vi "rsidr_core_global.vi"() -> ()   [LabVIEW 2020, in "Rohde&Schwarz CMWXP NR FR1 Measurement.lvlib"] (continued)
emission measurements exceeding the specified spectrum emission mask limits.\nDefault unit:  % \n\n<MarginX>\n float\nX-position of the margin of an area\nDefault unit:  Hz \n\n<MarginY>\n float\nY-value of the margin of an area\nDefault unit:  dB\n\nAvailable Repeated Capabilities:\ninstance: i0, i1, i2, i3, i4, i5, i6, i7, i8, i9, i10, i11, i12, i13, i14, i15, i16, i17, i18, i19, i20, i21, i22, i23, i24, i25, i26, i27, i28, i29, i30, i31, i32\r\n\nRemote-control command(s):\nFETCh:NRSub:MEAS<i>:MEValuation:SEMask:MARGin:MINimum:NEGativ?"}, {"Level"=4, "Class Only"=FALSE, "Identifier"="RSCMWXPNRFR1M_ATTR_FETCH_MULTI_EVAL_MEAS_SEM_MARGIN_ALL_RESULTS", "Descriptive Name"="Fetch Multi Eval Meas SEM Margin All Results", "Data Type"=enum."RawString", "Command"="FETC:NRS:MEAS{instance}:MEV:SEM:MARG:ALL?", "Access"=enum."Read Only", "Range Table"="", "Read Callback"="", "Write Callback"="", "Range Callback"="", "Check Callback"="", "Rngtable Callback"="", "Coerce Callback"="", "Supported Models"="", "Instrument Options"="", "Check Status Callback"="", "Flags"=0, "Help"="Returns spectrum emission mask margin results. A negative margin indicates that the trace is located above the limit line, i.e. the limit is exceeded. Results are provided for the current, average and maximum traces. For each trace, 24 values related to the negative (Neg) and positive (Pos) offset frequencies of emission mask areas 1 to 12 are provided. For inactive areas, NCAP is returned.\n\nReturn values:  \n<1_Reliability>\n decimal\n\n<2_OutOfTol>\n decimal\nOut of tolerance result, i.e. percentage of measurement intervals of the statistic count for spectrum emission measurements exceeding the specified spectrum emission mask limits.\nDefault unit:  % \n\n<3_CurrNeg1> ... <14_CurrNeg12>\n float\nMargin results for current trace, negative offsets\nDefault unit:  dB \n\n<15_CurrPos1> ... <26_CurrPos12>\n float\nMargin results for current trace, positive offsets\nDefault unit:  dB \n\n<27_AvgNeg1> ... <38_AvgNeg12>\n float\nMargin results for average trace, negative offsets\nDefault unit:  dB \n\n<39_AvgPos1> ... <50_AvgPos12>\n float\nMargin results for average trace, positive offsets\nDefault unit:  dB \n\n<51_MinNeg1> ... <62_MinNeg12>\n float\nMargin results for maximum trace (resulting in minimum margins), negative offsets\nDefault unit:  dB \n\n<63_MinPos1> ... <74_MinPos12>\n float\nMargin results for maximum trace (resulting in minimum margins), positive offsets\nDefault unit:  dB\n\nAvailable Repeated Capabilities:\ninstance: i0, i1, i2, i3, i4, i5, i6, i7, i8, i9, i10, i11, i12, i13, i14, i15, i16, i17, i18, i19, i20, i21, i22, i23, i24, i25, i26, i27, i28, i29, i30, i31, i32\r\n\nRemote-control command(s):\nFETCh:NRSub:MEAS<i>:MEValuation:SEMask:MARGin:ALL?"}, {"Level"=4, "Class Only"=TRUE, "Identifier"="", "Descriptive Name"="RBW Trace", "Data Type"=enum."ViInt32", "Command"="", "Access"=enum."Read Only", "Range Table"="", "Read Callback"="", "Write Callback"="", "Range Callback"="", "Check Callback"="", "Rngtable Callback"="", "Coerce Callback"="", "Supported Models"="", "Instrument Options"="", "Check Status Callback"="", "Flags"=0, "Help"="This class contains commands to fetch trace results for the individual resolution bandwidths."}, {"Level"=5, "Class Only"=FALSE, "Identifier"="RSCMWXPNRFR1M_ATTR_READ_MULTI_EVAL_MEAS_SEM_TRACE_RBW_CURRENT_RESULTS", "Descriptive Name"="Read Multi Eval Meas SEM Trace RBW Current Results", "Data Type"=enum."RawString", "Command"="READ:NRS:MEAS{instance}:MEV:TRAC:SEM:RBW{RBW}:CURR?", "Access"=enum."Read Only", "Range Table"="", "Read Callback"="", "Write Callback"="", "Range Callback"="", "Check Callback"="", "Rngtable Callback"="", "Coerce Callback"="", "Supported Models"="", "Instrument Options"="", "Check Status Callback"="", "Flags"=0, "Help"="Returns the values of the spectrum emission traces. Separate traces are available for the individual resolution bandwidths (<kHz>). The results of the current trace are returned.\n\nReturn values:\n<Reliability>\n decimal\n\n<Power>\n float\nComma-separated list of power results\nThe value in the middle of the result array corresponds to the center frequency. The test point separation between two results depends on the resolution bandwidth. If there is no result for a frequency because no limit is defined, INV is returned.\nDefault unit:  dBm\n\nAvailable Repeated Capabilities:\ninstance: i0, i1, i2, i3, i4, i5, i6, i7, i8, i9, i10, i11, i12, i13, i14, i15, i16, i17, i18, i19, i20, i21, i22, i23, i24, i25, i26, i27, i28, i29, i30, i31, i32\r\nRBW: kHz30, kHz100, MHz1, BW1Pc, BW2Pc\r\n\nRemote-control command(s):\nREAD:NRSub:MEAS<i>:MEValuation:TRACe:SEMask:RBW<kHz>:CURRent?"}, {"Level"=5, "Class Only"=FALSE, "Identifier"="RSCMWXPNRFR1M_ATTR_READ_MULTI_EVAL_MEAS_SEM_TRACE_RBW_AVERAGE_RESULTS", "Descriptive Name"="Read Multi Eval Meas SEM Trace RBW Average Results", "Data Type"=enum."RawString", "Command"="READ:NRS:MEAS{instance}:MEV:TRAC:SEM:RBW{RBW}:AVER?", "Access"=enum."Read Only", "Range Table"="", "Read Callback"="", "Write Callback"="", "Range Callback"="", "Check Callback"="", "Rngtable Callback"="", "Coerce Callback"="", "Supported Models"="", "Instrument Options"="", "Check Status Callback"="", "Flags"=0, "Help"="Returns the values of the spectrum emission traces. Separate traces are available for the individual resolution bandwidths (<kHz>). The results of the average trace are returned.\n\nReturn values:\n<Reliability>\n decimal\n\n<Power>\n float\nComma-separated list of power results\nThe value in the middle of the result array corresponds to the center frequency. The test point separation between two results depends on the resolution bandwidth. If there is no result for a frequency because no limit is defined, INV is returned.\nDefault unit:  dBm\n\nAvailable Repeated Capabilities:\ninstance: i0, i1, i2, i3, i4, i5, i6, i7, i8, i9, i10, i11, i12, i13, i14, i15, i16, i17, i18, i19, i20, i21, i22, i23, i24, i25, i26, i27, i28, i29, i30, i31, i32\r\nRBW: kHz30, kHz100, MHz1, BW1Pc, BW2Pc\r\n\nRemote-control command(s):\nREAD:NRSub:MEAS<i>:MEValuation:TRACe:SEMask:RBW<kHz>:AVERage?"}, {"Level"=5, "Class Only"=FALSE, "Identifier"="RSCMWXPNRFR1M_ATTR_READ_MULTI_EVAL_MEAS_SEM_TRACE_RBW_MAXIMUM_RESULTS", "Descriptive Name"="Read Multi Eval Meas SEM Trace RBW Maximum Results", "Data Type"=enum."RawString", "Command"="READ:NRS:MEAS{instance}:MEV:TRAC:SEM:RBW{RBW}:MAX?", "Access"=enum."Read Only", "Range Table"="", "Read Callback"="", "Write Callback"="", "Range Callback"="", "Check Callback"="", "Rngtable Callback"="", "Coerce Callback"="", "Supported Models"="", "Instrument Options"="", "Check Status Callback"="", "Flags"=0, "Help"="Returns the values of the spectrum emission traces. Separate traces are available for the individual resolution bandwidths (<kHz>). The results of the maximum trace are returned.\n\nReturn values:\n<Reliability>\n decimal\n\n<Power>\n float\nComma-separated list of power results\nThe value in the middle of the result array corresponds to the center frequency. The test point separation between two results depends on the resolution bandwidth. If there is no result for a frequency because no limit is defined, INV is returned.\nDefault unit:  dBm\n\nAvailable Repeated Capabilities:\ninstance: i0, i1, i2, i3, i4, i5, i6, i7, i8, i9, i10, i11, i12, i13, i14, i15, i16, i17, i18, i19, i20, i21, i22, i23, i24, i25, i26, i27, i28, i29, i30, i31, i32\r\nRBW: kHz30, kHz100, MHz1, BW1Pc, BW2Pc\r\n\nRemote-control command(s):\nREAD:NRSub:MEAS<i>:MEValuation:TRACe:SEMask:RBW<kHz>:MAXimum?"}, {"Level"=5, "Class Only"=FALSE, "Identifier"="RSCMWXPNRFR1M_ATTR_FETCH_MULTI_EVAL_MEAS_SEM_TRACE_RBW_CURRENT_RESULTS", "Descriptive Name"="Fetch Multi Eval Meas SEM Trace RBW Current Results", "Data Type"=enum."RawString", "Command"="FETC:NRS:MEAS{instance}:MEV:TRAC:SEM:RBW{RBW}:CURR?", "Access"=enum."Read Only", "Range Table"="", "Read Callback"="", "Write Callback"="", "Range Callback"="", "Check Callback"="", "Rngtable Callback"="", "Coerce Callback"="", "Supported Models"="", "Instrument Options"="", "Check Status Callback"="", "Flags"=0, "Help"="Returns the values of the spectrum emission traces. Separate traces are available for the individual resolution bandwidths (<kHz>). The results of the current trace are returned.\n\nReturn values:\n<Reliability>\n decimal\n\n<Power>\n float\nComma-separated list of power results\nThe value in the middle of the result array corresponds to the center frequency. The test point separation between two results depends on the resolution bandwidth. If there is no result for a frequency because no limit is defined, INV is returned.\nDefault unit:  dBm\n\nAvailable Repeated Capabilities:\ninstance: i0, i1, i2, i3, i4, i5, i6, i7, i8, i9, i10, i11, i12, i13, i14, i15, i16, i17, i18, i19, i20, i21, i22, i23, i24, i25, i26, i27, i28, i29, i30, i31, i32\r\nRBW: kHz30, kHz100, MHz1, BW1Pc, BW2Pc\r\n\nRemote-control command(s):\nFETCh:NRSub:MEAS<i>:MEValuation:TRACe:SEMask:RBW<kHz>:CURRent?"}, {"Level"=5, "Class Only"=FALSE, "Identifier"="RSCMWXPNRFR1M_ATTR_FETCH_MULTI_EVAL_MEAS_SEM_TRACE_RBW_AVERAGE_RESULTS", "Descriptive Name"="Fetch Multi Eval Meas SEM Trace RBW Average Results", "Data Type"=enum."RawString", "Command"="FETC:NRS:MEAS{instance}:MEV:TRAC:SEM:RBW{RBW}:AVER?", "Access"=enum."Read Only", "Range Table"="", "Read Callback"="", "Write Callback"="", "Range Callback"="", "Check Callback"="", "Rngtable Callback"="", "Coerce Callback"="", "Supported Models"="", "Instrument Options"="", "Check Status Callback"="", "Flags"=0, "Help"="Returns the values of the spectrum emission traces. Separate traces are available for the individual resolution bandwidths (<kHz>). The results of the average trace are returned.\n\nReturn values:\n<Reliability>\n decimal\n\n<Power>\n float\nComma-separated list of power results\nThe value in the middle of the result array corresponds to the center frequency. The test point separation between two results depends on the resolution bandwidth. If there is no result for a frequency because no limit is defined, INV is returned.\nDefault unit:  dBm\n\nAvailable Repeated Capabilities:\ninstance: i0, i1, i2, i3, i4, i5, i6, i7, i8, i9, i10, i11, i12, i13, i14, i15, i16, i17, i18, i19, i20, i21, i22, i23, i24, i25, i26, i27, i28, i29, i30, i31, i32\r\nRBW: kHz30, kHz100, MHz1, BW1Pc, BW2Pc\r\n\nRemote-control command(s):\nFETCh:NRSub:MEAS<i>:MEValuation:TRACe:SEMask:RBW<kHz>:AVERage?"}, {"Level"=5, "Class Only"=FALSE, "Identifier"="RSCMWXPNRFR1M_ATTR_FETCH_MULTI_EVAL_MEAS_SEM_TRACE_RBW_MAXIMUM_RESULTS", "Descriptive Name"="Fetch Multi Eval Meas SEM Trace RBW Maximum Results", "Data Type"=enum."RawString", "Command"="FETC:NRS:MEAS{instance}:MEV:TRAC:SEM:RBW{RBW}:MAX?", "Access"=enum."Read Only", "Range Table"="", "Read Callback"="", "Write Callback"="", "Range Callback"="", "Check Callback"="", "Rngtable Callback"="", "Coerce Callback"="", "Supported Models"="", "Instrument Options"="", "Check Status Callback"="", "Flags"=0, "Help"="Returns the values of the spectrum emission traces. Separate traces are available for the individual resolution bandwidths (<kHz>). The results of the maximum trace are returned.\n\nReturn values:\n<Reliability>\n decimal\n\n<Power>\n float\nComma-separated list of power results\nThe value in the middle of the result array corresponds to the center frequency. The test point separation between two results depends on the resolution bandwidth. If there is no result for a frequency because no limit is defined, INV is returned.\nDefault unit:  dBm\n\nAvailable Repeated Capabilities:\ninstance: i0, i1, i2, i3, i4, i5, i6, i7, i8, i9, i10, i11, i12, i13, i14, i15, i16, i17, i18, i19, i20, i21, i22, i23, i24, i25, i26, i27, i28, i29, i30, i31, i32\r\nRBW: kHz30, kHz100, MHz1, BW1Pc, BW2Pc\r\n\nRemote-control command(s):\nFETCh:NRSub:MEAS<i>:MEValuation:TRACe:SEMask:RBW<kHz>:MAXimum?"}, {"Level"=4, "Class Only"=TRUE, "Identifier"="", "Descriptive Name"="Area Trace", "Data Type"=enum."ViInt32", "Command"="", "Access"=enum."Read Only", "Range Table"="", "Read Callback"="", "Write Callback"="", "Range Callback"="", "Check Callback"="", "Rngtable Callback"="", "Coerce Callback"="", "Supported Models"="", "Instrument Options"="", "Check Status Callback"="", "Flags"=0, "Help"="This class contains commands to fetch trace results for specific spectrum emission mask areas."}, {"Level"=5, "Class Only"=FALSE, "Identifier"="RSCMWXPNRFR1M_ATTR_FETCH_MULTI_EVAL_MEAS_SEM_AREA_POSITIVE_CURRENT_RESULTS", "Descriptive Name"="Fetch Multi Eval Meas SEM Trace Area Positive Current Results", "Data Type"=enum."RawString", "Command"="FETC:NRS:MEAS{instance}:MEV:TRAC:SEM:AREA{Area}:POS:CURR?", "Access"=enum."Read Only", "Range Table"="", "Read Callback"="", "Write Callback"="", "Range Callback"="", "Check Callback"="", "Rngtable Callback"="", "Coerce Callback"="", "Supported Models"="", "Instrument Options"="", "Check Status Callback"="", "Flags"=0, "Help"="Returns the measured power values for a single spectrum emission mask area with enabled limit check. The results of the current trace above (Positive) the carrier center frequency are returned.\n\nReturn values:\n<Reliability>\n decimal\n\n<RBW>\n K030 | K100 | M1 | PC1 | PC2\nUsed resolution bandwidth (configured via limit settings).\nK030: RBW 30 kHz\nK100: RBW 100 kHz\nM1: RBW 1 MHz\nPC1: RBW 1 % of channel BW\nPC2: RBW 2 % of channel BW\n\n<Power>\n float\nComma-separated list of power results\nIf the limit check is disabled for the area, INV is returned.\nDefault unit:  dBm\n\nAvailable Repeated Capabilities:\ninstance: i0, i1, i2, i3, i4, i5, i6, i7, i8, i9, i10, i11, i12, i13, i14, i15, i16, i17, i18, i19, i20, i21, i22, i23, i24, i25, i26, i27, i28, i29, i30, i31, i32\r\nArea: a1, a2, a3, a4, a5, a6, a7, a8, a9, a10, a11, a12\r\n\nRemote-control command(s):\nFETCh:NRSub:MEAS<i>:MEValuation:TRACe:SEMask:AREA<area>:POSitive:CURRent?"}, {"Level"=5, "Class Only"=FALSE, "Identifier"="RSCMWXPNRFR1M_ATTR_FETCH_MULTI_EVAL_MEAS_SEM_AREA_POSITIVE_AVERAGE_RESULTS", "Descriptive Name"="Fetch Multi Eval Meas SEM Trace Area Positive Average Results", "Data Type"=enum."RawString", "Command"="FETC:NRS:MEAS{instance}:MEV:TRAC:SEM:AREA{Area}:POS:AVER?", "Access"=enum."Read Only", "Range Table"="", "Read Callback"="", "Write Callback"="", "Range Callback"="", "Check Callback"="", "Rngtable Callback"="", "Coerce Callback"="", "Supported Models"="", "Instrument Options"="", "Check Status Callback"="", "Flags"=0, "Help"="Returns the measured power values for a single spectrum emission mask area with enabled limit check. The results of the average  trace above (Positive) the carrier center frequency are returned.\n\n\nReturn values:\n<Reliability>\n decimal\n\n<RBW>\n K030 | K100 | M1 | PC1 | PC2\nUsed resolution bandwidth (configured via limit settings).\nK030: RBW 30 kHz\nK100: RBW 100 kHz\nM1: RBW 1 MHz\nPC1: RBW 1 % of channel BW\nPC2: RBW 2 % of channel BW\n\n<Power>\n float\nComma-separated list of power results\nIf the limit check is disabled for the area, INV is returned.\nDefault unit:  dBm\n\nAvailable Repeated Capabilities:\ninstance: i0, i1, i2, i3, i4, i5, i6, i7, i8, i9, i10, i11, i12, i13, i14, i15, i16, i17, i18, i19, i20, i21, i22, i23, i24, i25, i26, i27, i28, i29, i30, i31, i32\r\nArea: a1, a2, a3, a4, a5, a6, a7, a8, a9, a10, a11, a12\r\n\nRemote-control command(s):\nFETCh:NRSub:MEAS<i>:MEValuation:TRACe:SEMask:AREA<area>:POSitive:AVERage?"}, {"Level"=5, "Class Only"=FALSE, "Identifier"="RSCMWXPNRFR1M_ATTR_FETCH_MULTI_EVAL_MEAS_SEM_AREA_POSITIVE_MAXIMUM_RESULTS", "Descriptive Name"="Fetch Multi Eval Meas SEM Trace Area Positive Maximum Results", "Data Type"=enum."RawString", "Command"="FETC:NRS:MEAS{instance}:MEV:TRAC:SEM:AREA{Area}:POS:MAX?", "Access"=enum."Read Only", "Range Table"="", "Read Callback"="", "Write Callback"="", "Range Callback"="", "Check Callback"="", "Rngtable Callback"="", "Coerce Callback"="", "Supported Models"="", "Instrument Options"="", "Check Status Callback"="", "Flags"=0, "Help"="Returns the measured power values for a single spectrum emission mask area with enabled limit check. The results of the maximum trace above (Positive) the carrier center frequency are returned.\n\n\nReturn values:\n<Reliability>\n decimal\n\n<RBW>\n K030 | K100 | M1 | PC1 | PC2\nUsed resolution bandwidth (configured via limit settings).\nK030: RBW 30 kHz\nK100: RBW 100 kHz\nM1: RBW 1 MHz\nPC1: RBW 1 % of channel BW\nPC2: RBW 2 % of channel BW\n\n<Power>\n float\nComma-separated list of power results\nIf the limit check is disabled for the area, INV is returned.\nDefault unit:  dBm\n\nAvailable Repeated Capabilities:\ninstance: i0, i1, i2, i3, i4, i5, i6, i7, i8, i9, i10, i11, i12, i13, i14, i15, i16, i17, i18, i19, i20, i21, i22, i23, i24, i25, i26, i27, i28, i29, i30, i31, i32\r\nArea: a1, a2, a3, a4, a5, a6, a7, a8, a9, a10, a11, a12\r\n\nRemote-control command(s):\nFETCh:NRSub:MEAS<i>:MEValuation:TRACe:SEMask:AREA<area>:POSitive:MAXimum?"}, {"Level"=5, "Class Only"=FALSE, "Identifier"="RSCMWXPNRFR1M_ATTR_FETCH_MULTI_EVAL_MEAS_SEM_AREA_NEGATIVE_CURRENT_RESULTS", "Descriptive Name"="Fetch Multi Eval Meas SEM Trace Area Negative Current Results", "Data Type"=enum."RawString", "Command"="FETC:NRS:MEAS{instance}:MEV:TRAC:SEM:AREA{Area}:NEG:CURR?", "Access"=enum."Read Only", "Range Table"="", "Read Callback"="", "Write Callback"="", "Range Callback"="", "Check Callback"="", "Rngtable Callback"="", "Coerce Callback"="", "Supported Models"="", "Instrument Options"="", "Check Status Callback"="", "Flags"=0, "Help"="Returns the measured power values for a single spectrum emission mask area with enabled limit check.The results of the current trace below (Negative) the carrier center frequency are returned.\n\nReturn values:\n<Reliability>\n decimal\n\n<RBW>\n K030 | K100 | M1 | PC1 | PC2\nUsed resolution bandwidth (configured via limit settings).\nK030: RBW 30 kHz\nK100: RBW 100 kHz\nM1: RBW 1 MHz\nPC1: RBW 1 % of channel BW\nPC2: RBW 2 % of channel BW\n\n<Power>\n float\nComma-separated list of power results\nIf the limit check is disabled for the area, INV is returned.\nDefault unit:  dBm\n\nAvailable Repeated Capabilities:\ninstance: i0, i1, i2, i3, i4, i5, i6, i7, i8, i9, i10, i11, i12, i13, i14, i15, i16, i17, i18, i19, i20, i21, i22, i23, i24, i25, i26, i27, i28, i29, i30, i31, i32\r\nArea: a1, a2, a3, a4, a5, a6, a7, a8, a9, a10, a11, a12\r\n\nRemote-control command(s):\nFETCh:NRSub:MEAS<i>:MEValuation:TRACe:SEMask:AREA<area>:NEGative:CURRent?"}, {"Level"=5, "Class Only"=FALSE, "Identifier"="RSCMWXPNRFR1M_ATTR_FETCH_MULTI_EVAL_MEAS_SEM_AREA_NEGATIVE_AVERAGE_RESULTS", "Descriptive Name"="Fetch Multi Eval Meas SEM Trace Area Negative Average Results", "Data Type"=enum."RawString", "Command"="FETC:NRS:MEAS{instance}:MEV:TRAC:SEM:AREA{Area}:NEG:AVER?", "Access"=enum."Read Only", "Range Table"="", "Read Callback"="", "Write Callback"="", "Range Callback"="", "Check Callback"="", "Rngtable Callback"="", "Coerce Callback"="", "Supported Models"="", "Instrument Options"="", "Check Status Callback"="", "Flags"=0, "Help"="Returns the measured power values for a single spectrum emission mask area with enabled limit check.The results of the average  trace below (Negative) the carrier center frequency are returned.\n\nReturn values:\n<Reliability>\n decimal\n\n<RBW>\n K030 | K100 | M1 | PC1 | PC2\nUsed resolution bandwidth (configured via limit settings).\nK030: RBW 30 kHz\nK100: RBW 100 kHz\nM1: RBW 1 MHz\nPC1: RBW 1 % of channel BW\nPC2: RBW 2 % of channel BW\n\n<Power>\n float\nComma-separated list of power results\nIf the limit check is disabled for the area, INV is returned.\nDefault unit:  dBm\n\nAvailable Repeated Capabilities:\ninstance: i0, i1, i2, i3, i4, i5, i6, i7, i8, i9, i10, i11, i12, i13, i14, i15, i16, i17, i18, i19, i20, i21, i22, i23, i24, i25, i26, i27, i28, i29, i30, i31, i32\r\nArea: a1, a2, a3, a4, a5, a6, a7, a8, a9, a10, a11, a12\r\n\nRemote-control command(s):\nFETCh:NRSub:MEAS<i>:MEValuation:TRACe:SEMask:AREA<area>:NEGative:AVERage?"}, {"Level"=5, "Class Only"=FALSE, "Identifier"="RSCMWXPNRFR1M_ATTR_FETCH_MULTI_EVAL_MEAS_SEM_AREA_NEGATIVE_MAXIMUM_RESULTS", "Descriptive Name"="Fetch Multi Eval Meas SEM Trace Area Negative Maximum Results", "Data Type"=enum."RawString", "Command"="FETC:NRS:MEAS{instance}:MEV:TRAC:SEM:AREA{Area}:NEG:MAX?", "Access"=enum."Read Only", "Range Table"="", "Read Callback"="", "Write Callback"="", "Range Callback"="", "Check Callback"="", "Rngtable Callback"="", "Coerce Callback"="", "Supported Models"="", "Instrument Options"="", "Check Status Callback"="", "Flags"=0, "Help"="Returns the measured power values for a single spectrum emission mask area with enabled limit check. The results of the maximum trace below (Negative) the carrier center frequency are returned.\n\nReturn values:\n<Reliability>\n decimal\n\n<RBW>\n K030 | K100 | M1 | PC1 | PC2\nUsed resolution bandwidth (configured via limit settings).\nK030: RBW 30 kHz\nK100: RBW 100 kHz\nM1: RBW 1 MHz\nPC1: RBW 1 % of channel BW\nPC2: RBW 2 % of channel BW\n\n<Power>\n float\nComma-separated list of power results\nIf the limit check is disabled for the area, INV is returned.\nDefault unit:  dBm\n\nAvailable Repeated Capabilities:\ninstance: i0, i1, i2, i3, i4, i5, i6, i7, i8, i9, i10, i11, i12, i13, i14, i15, i16, i17, i18, i19, i20, i21, i22, i23, i24, i25, i26, i27, i28, i29, i30, i31, i32\r\nArea: a1, a2, a3, a4, a5, a6, a7, a8, a9, a10, a11, a12\r\n\nRemote-control command(s):\nFETCh:NRSub:MEAS<i>:MEValuation:TRACe:SEMask:AREA<area>:NEGative:MAXimum?"}, {"Level"=5, "Class Only"=FALSE, "Identifier"="RSCMWXPNRFR1M_ATTR_FETCH_MULTI_EVAL_MEAS_SEM_TRACE_AREA_POSITIVE_FREQUENCIES", "Descriptive Name"="Fetch Multi Eval Meas SEM Trace Area Positive Frequencies", "Data Type"=enum."RawString", "Command"="FETC:NRS:MEAS{instance}:MEV:TRAC:SEM:AREA{Area}:POS:FREQ?", "Access"=enum."Read Only", "Range Table"="", "Read Callback"="", "Write Callback"="", "Range Callback"="", "Check Callback"="", "Rngtable Callback"="", "Coerce Callback"="", "Supported Models"="", "Instrument Options"="", "Check Status Callback"="", "Flags"=0, "Help"="Returns the frequencies of a single spectrum emission mask area. The area is located above (Positive) the carrier center frequency. At the returned frequencies, the power values are measured.\n\nReturn values:\n<Reliability>\n decimal\n\n<RBW>\n K030 | K100 | M1 | PC1 | PC2\nUsed resolution bandwidth (configured via limit settings).\nK030: RBW 30 kHz\nK100: RBW 100 kHz\nM1: RBW 1 MHz\nPC1: RBW 1 % of channel BW\nPC2: RBW 2 % of channel BW\n\n<Frequency>\n float\nComma-separated list of frequency values\nDefault unit:  Hz\n\nAvailable Repeated Capabilities:\ninstance: i0, i1, i2, i3, i4, i5, i6, i7, i8, i9, i10, i11, i12, i13, i14, i15, i16, i17, i18, i19, i20, i21, i22, i23, i24, i25, i26, i27, i28, i29, i30, i31, i32\r\nArea: a1, a2, a3, a4, a5, a6, a7, a8, a9, a10, a11, a12\r\n\nRemote-control command(s):\nFETCh:NRSub:MEAS<i>:MEValuation:TRACe:SEMask:AREA<area>:POSitive:FREQuency?"}, {"Level"=5, "Class Only"=FALSE, "Identifier"="RSCMWXPNRFR1M_ATTR_FETCH_MULTI_EVAL_MEAS_SEM_TRACE_AREA_NEGATIVE_FREQUENCIES", "Descriptive Name"="Fetch Multi Eval Meas SEM Trace Area Negative Frequencies", "Data Type"=enum."RawString", "Command"="FETC:NRS:MEAS{instance}:MEV:TRAC:SEM:AREA{Area}:NEG:FREQ?", "Access"=enum."Read Only", "Range Table"="", "Read Callback"="", "Write Callback"="", "Range Callback"="", "Check Callback"="", "Rngtable Callback"="", "Coerce Callback"="", "Supported Models"="", "Instrument Options"="", "Check Status Callback"="", "Flags"=0, "Help"="Returns the frequencies of a single spectrum emission mask area. The area is located below (Negative) the carrier center frequency. At the returned frequencies, the power values are measured.\n\nReturn values:\n<Reliability>\n decimal\n\n<RBW>\n K030 | K100 | M1 | PC1 | PC2\nUsed resolution bandwidth (configured via limit settings).\nK030: RBW 30 kHz\nK100: RBW 100 kHz\nM1: RBW 1 MHz\nPC1: RBW 1 % of channel BW\nPC2: RBW 2 % of channel BW\n\n<Frequency>\n float\nComma-separated list of frequency values\nDefault unit:  Hz\n\nAvailable Repeated Capabilities:\ninstance: i0, i1, i2, i3, i4, i5, i6, i7, i8, i9, i10, i11, i12, i13, i14, i15, i16, i17, i18, i19, i20, i21, i22, i23, i24, i25, i26, i27, i28, i29, i30, i31, i32\r\nArea: a1, a2, a3, a4, a5, a6, a7, a8, a9, a10, a11, a12\r\n\nRemote-control command(s):\nFETCh:NRSub:MEAS<i>:MEValuation:TRACe:SEMask:AREA<area>:NEGative:FREQuency?"}, {"Level"=3, "Class Only"=TRUE, "Identifier"="", "Descriptive Name"="ACLR Spectrum", "Data Type"=enum."ViInt32", "Command"="", "Access"=enum."Read Only", "Range Table"="", "Read Callback"="", "Write Callback"="", "Range Callback"="", "Check Callback"="", "Rngtable Callback"="", "Coerce Callback"="", "Supported Models"="", "Instrument Options"="", "Check Status Callback"="", "Flags"=0, "Help"="The commands in thie class return the ACLR spectrum results."}, {"Level"=4, "Class Only"=FALSE, "Identifier"="RSCMWXPNRFR1M_ATTR_READ_MULTI_EVAL_MEAS_TRACE_ACLR_CURRENT_RESULTS", "Descriptive Name"="Read Multi Eval Meas Trace ACLR Current Results", "Data Type"=enum."RawString", "Command"="READ:NRS:MEAS{instance}:MEV:TRAC:ACLR:CURR?", "Access"=enum."Read Only", "Range Table"="", "Read Callback"="", "Write Callback"="", "Range Callback"="", "Check Callback"="", "Rngtable Callback"="", "Coerce Callback"="", "Supported Models"="", "Instrument Options"="", "Check Status Callback"="", "Flags"=0, "Help"="Returns the absolute powers as displayed in the ACLR diagram for NR standalone. The current values are retrieved.\n\nReturn values:  \n<Reliability>\n decimal\n\n<UTRA2neg>\n float\nPower in the second UTRA channel with lower frequency\nDefault unit:  dBm \n\n<UTRA1neg>\n float\nPower in the first UTRA channel with lower frequency\nDefault unit:  dBm \n\n<NRneg>\n float\nPower in the first NR channel with lower frequency\nDefault unit:  dBm \n\n<Carrier>\n float\nPower in the allocated NR channel\nDefault unit:  dBm \n\n<NRpos>\n float\nPower in the first NR channel with higher frequency\nDefault unit:  dBm \n\n<UTRA1pos>\n float\nPower in the first UTRA channel with higher frequency\nDefault unit:  dBm \n\n<UTRA2pos>\n float\nPower in the second UTRA channel with higher frequency\nDefault unit:  dBm\n\nAvailable Repeated Capabilities:\ninstance: i0, i1, i2, i3, i4, i5, i6, i7, i8, i9, i10, i11, i12, i13, i14, i15, i16, i17, i18, i19, i20, i21, i22, i23, i24, i25, i26, i27, i28, i29, i30, i31, i32\r\n\nRemote-control command(s):\nREAD:NRSub:MEAS<i>:MEValuation:TRACe:ACLR:CURRent?"}, {"Level"=4, "Class Only"=FALSE, "Identifier"="RSCMWXPNRFR1M_ATTR_READ_MULTI_EVAL_MEAS_TRACE_ACLR_AVERAGE_RESULTS", "Descriptive Name"="Read Multi Eval Meas Trace ACLR Average Results", "Data Type"=enum."RawString", "Command"="READ:NRS:MEAS{instance}:MEV:TRAC:ACLR:AVER?", "Access"=enum."Read Only", "Range Table"="", "Read Callback"="", "Write Callback"="", "Range Callback"="", "Check Callback"="", "Rngtable Callback"="", "Coerce Callback"="", "Supported Models"="", "Instrument Options"="", "Check Status Callback"="", "Flags"=0, "Help"="Returns the absolute powers as displayed in the ACLR diagram for NR standalone. The average values are retrieved.\n\nReturn values:  \n<Reliability>\n decimal\n\n<UTRA2neg>\n float\nPower in the second UTRA channel with lower frequency\nDefault unit:  dBm \n\n<UTRA1neg>\n float\nPower in the first UTRA channel with lower frequency\nDefault unit:  dBm \n\n<NRneg>\n float\nPower in the first NR channel with lower frequency\nDefault unit:  dBm \n\n<Carrier>\n float\nPower in the allocated NR channel\nDefault unit:  dBm \n\n<NRpos>\n float\nPower in the first NR channel with higher frequency\nDefault unit:  dBm \n\n<UTRA1pos>\n float\nPower in the first UTRA channel with higher frequency\nDefault unit:  dBm \n\n<UTRA2pos>\n float\nPower in the second UTRA channel with higher frequency\nDefault unit:  dBm\n\nAvailable Repeated Capabilities:\ninstance: i0, i1, i2, i3, i4, i5, i6, i7, i8, i9, i10, i11, i12, i13, i14, i15, i16, i17, i18, i19, i20, i21, i22, i23, i24, i25, i26, i27, i28, i29, i30, i31, i32\r\n\nRemote-control command(s):\nREAD:NRSub:MEAS<i>:MEValuation:TRACe:ACLR:AVERage?"}, {"Level"=4, "Class Only"=FALSE, "Identifier"="RSCMWXPNRFR1M_ATTR_FETCH_MULTI_EVAL_MEAS_TRACE_ACLR_CURRENT_RESULTS", "Descriptive Name"="Fetch Multi Eval Meas Trace ACLR Current Results", "Data Type"=enum."RawString", "Command"="FETC:NRS:MEAS{instance}:MEV:TRAC:ACLR:CURR?", "Access"=enum."Read Only", "Range Table"="", "Read Callback"="", "Write Callback"="", "Range Callback"="", "Check Callback"="", "Rngtable Callback"="", "Coerce Callback"="", "Supported Models"="", "Instrument Options"="", "Check Status Callback"="", "Flags"=0, "Help"="Returns the absolute powers as displayed in the ACLR diagram for NR standalone. The current values are retrieved.\n\nReturn values:  \n<Reliability>\n decimal\n\n<UTRA2neg>\n float\nPower in the second UTRA channel with lower frequency\nDefault unit:  dBm \n\n<UTRA1neg>\n float\nPower in the first UTRA channel with lower frequency\nDefault unit:  dBm \n\n<NRneg>\n float\nPower in the first NR channel with lower frequency\nDefault unit:  dBm \n\n<Carrier>\n float\nPower in the allocated NR channel\nDefault unit:  dBm \n\n<NRpos>\n float\nPower in the first NR channel with higher frequency\nDefault unit:  dBm \n\n<UTRA1pos>\n float\nPower in the first UTRA channel with higher frequency\nDefault unit:  dBm \n\n<UTRA2pos>\n float\nPower in the second UTRA channel with higher frequency\nDefault unit:  dBm\n\nAvailable Repeated Capabilities:\ninstance: i0, i1, i2, i3, i4, i5, i6, i7, i8, i9, i10, i11, i12, i13, i14, i15, i16, i17, i18, i19, i20, i21, i22, i23, i24, i25, i26, i27, i28, i29, i30, i31, i32\r\n\nRemote-control command(s):\nFETCh:NRSub:MEAS<i>:MEValuation:TRACe:ACLR:CURRent?"}, {"Level"=4, "Class Only"=FALSE, "Identifier"="RSCMWXPNRFR1M_ATTR_FETCH_MULTI_EVAL_MEAS_TRACE_ACLR_AVERAGE_RESULTS", "Descriptive Name"="Fetch Multi Eval Meas Trace ACLR Average Results", "Data Type"=enum."RawString", "Command"="FETC:NRS:MEAS{instance}:MEV:TRAC:ACLR:AVER?", "Access"=enum."Read Only", "Range Table"="", "Read Callback"="", "Write Callback"="", "Range Callback"="", "Check Callback"="", "Rngtable Callback"="", "Coerce Callback"="", "Supported Models"="", "Instrument Options"="", "Check Status Callback"="", "Flags"=0, "Help"="Returns the absolute powers as displayed in the ACLR diagram for NR standalone. The average values are retrieved.\n\nReturn values:  \n<Reliability>\n decimal\n\n<UTRA2neg>\n float\nPower in the second UTRA channel with lower frequency\nDefault unit:  dBm \n\n<UTRA1neg>\n float\nPower in the first UTRA channel with lower frequency\nDefault unit:  dBm \n\n<NRneg>\n float\nPower in the first NR channel with lower frequency\nDefault unit:  dBm \n\n<Carrier>\n float\nPower in the allocated NR channel\nDefault unit:  dBm \n\n<NRpos>\n float\nPower in the first NR channel with higher frequency\nDefault unit:  dBm \n\n<UTRA1pos>\n float\nPower in the first UTRA channel with higher frequency\nDefault unit:  dBm \n\n<UTRA2pos>\n float\nPower in the second UTRA channel with higher frequency\nDefault unit:  dBm\n\nAvailable Repeated Capabilities:\ninstance: i0, i1, i2, i3, i4, i5, i6, i7, i8, i9, i10, i11, i12, i13, i14, i15, i16, i17, i18, i19, i20, i21, i22, i23, i24, i25, i26, i27, i28, i29, i30, i31, i32\r\n\nRemote-control command(s):\nFETCh:NRSub:MEAS<i>:MEValuation:TRACe:ACLR:AVERage?"}, {"Level"=4, "Class Only"=FALSE, "Identifier"="RSCMWXPNRFR1M_ATTR_READ_MULTI_EVAL_MEAS_TRACE_ACLR_ENDC_CURRENT_RESULTS", "Descriptive Name"="Read Multi Eval Meas Trace ACLR EN-DC Current Results", "Data Type"=enum."RawString", "Command"="READ:NRS:MEAS{instance}:MEV:TRAC:ACLR:ENDC:CURR?", "Access"=enum."Read Only", "Range Table"="", "Read Callback"="", "Write Callback"="", "Range Callback"="", "Check Callback"="", "Rngtable Callback"="", "Coerce Callback"="", "Supported Models"="", "Instrument Options"="", "Check Status Callback"="", "Flags"=0, "Help"="Returns the absolute powers as displayed in the ACLR diagram for EN-DC. The current values are retrieved.\n\nReturn values:  \n<Reliability>\n decimal\n\n<ENDCneg>\n float\nPower in the adjacent channel with lower frequency\nDefault unit:  dB \n\n<Carrier>\n float\nPower in the allocated channel (aggregated BW)\nDefault unit:  dBm \n\n<ENDCpos>\n float\nPower in the adjacent channel with higher frequency\nDefault unit:  dB\n\nAvailable Repeated Capabilities:\ninstance: i0, i1, i2, i3, i4, i5, i6, i7, i8, i9, i10, i11, i12, i13, i14, i15, i16, i17, i18, i19, i20, i21, i22, i23, i24, i25, i26, i27, i28, i29, i30, i31, i32\r\n\nRemote-control command(s):\nREAD:NRSub:MEAS<i>:MEValuation:TRACe:ACLR:ENDC:CURRent?"}, {"Level"=4, "Class Only"=FALSE, "Identifier"="RSCMWXPNRFR1M_ATTR_READ_MULTI_EVAL_MEAS_TRACE_ACLR_ENDC_AVERAGE_RESULTS", "Descriptive Name"="Read Multi Eval Meas Trace ACLR EN-DC Average Results", "Data Type"=enum."RawString", "Command"="READ:NRS:MEAS{instance}:MEV:TRAC:ACLR:ENDC:AVER?", "Access"=enum."Read Only", "Range Table"="", "Read Callback"="", "Write Callback"="", "Range Callback"="", "Check Callback"="", "Rngtable Callback"="", "Coerce Callback"="", "Supported Models"="", "Instrument Options"="", "Check Status Callback"="", "Flags"=0, "Help"="Returns the absolute powers as displayed in the ACLR diagram for EN-DC. The average values are retrieved.\n\nReturn values:  \n<Reliability>\n decimal\n\n<ENDCneg>\n float\nPower in the adjacent channel with lower frequency\nDefault unit:  dB \n\n<Carrier>\n float\nPower in the allocated channel (aggregated BW)\nDefault unit:  dBm \n\n<ENDCpos>\n float\nPower in the adjacent channel with higher frequency\nDefault unit:  dB\n\nAvailable Repeated Capabilities:\ninstance: i0, i1, i2, i3, i4, i5, i6, i7, i8, i9, i10, i11, i12, i13, i14, i15, i16, i17, i18, i19, i20, i21, i22, i23, i24, i25, i26, i27, i28, i29, i30, i31, i32\r\n\nRemote-control command(s):\nREAD:NRSub:MEAS<i>:MEValuation:TRACe:ACLR:ENDC:AVERage?"}, {"Level"=4, "Class Only"=FALSE, "Identifier"="RSCMWXPNRFR1M_ATTR_FETCH_MULTI_EVAL_MEAS_TRACE_ACLR_ENDC_CURRENT_RESULTS", "Descriptive Name"="Fetch Multi Eval Meas Trace ACLR EN-DC Current Results", "Data Type"=enum."RawString", "Command"="FETC:NRS:MEAS{instance}:MEV:TRAC:ACLR:ENDC:CURR?", "Access"=enum."Read Only", "Range Table"="", "Read Callback"="", "Write Callback"="", "Range Callback"="", "Check Callback"="", "Rngtable Callback"="", "Coerce Callback"="", "Supported Models"="", "Instrument Options"="", "Check Status Callback"="", "Flags"=0, "Help"="Returns the absolute powers as displayed in the ACLR diagram for EN-DC. The current values are retrieved.\n\nReturn values:  \n<Reliability>\n decimal\n\n<ENDCneg>\n float\nPower in the adjacent channel with lower frequency\nDefault unit:  dB \n\n<Carrier>\n float\nPower in the allocated channel (aggregated BW)\nDefault unit:  dBm \n\n<ENDCpos>\n float\nPower in the adjacent channel with higher frequency\nDefault unit:  dB\n\nAvailable Repeated Capabilities:\ninstance: i0, i1, i2, i3, i4, i5, i6, i7, i8, i9, i10, i11, i12, i13, i14, i15, i16, i17, i18, i19, i20, i21, i22, i23, i24, i25, i26, i27, i28, i29, i30, i31, i32\r\n\nRemote-control command(s):\nFETCh:NRSub:MEAS<i>:MEValuation:TRACe:ACLR:ENDC:CURRent?"}, {"Level"=4, "Class Only"=FALSE, "Identifier"="RSCMWXPNRFR1M_ATTR_FETCH_MULTI_EVAL_MEAS_TRACE_ACLR_ENDC_AVERAGE_RESULTS", "Descriptive Name"="Fetch Multi Eval Meas Trace ACLR EN-DC Average Results", "Data Type"=enum."RawString", "Command"="FETC:NRS:MEAS{instance}:MEV:TRAC:ACLR:ENDC:AVER?", "Access"=enum."Read Only", "Range Table"="", "Read Callback"="", "Write Callback"="", "Range Callback"="", "Check Callback"="", "Rngtable Callback"="", "Coerce Callback"="", "Supported Models"="", "Instrument Options"="", "Check Status Callback"="", "Flags"=0, "Help"="Returns the absolute powers as displayed in the ACLR diagram for EN-DC. The average values are retrieved.\n\nReturn values:  \n<Reliability>\n decimal\n\n<ENDCneg>\n float\nPower in the adjacent channel with lower frequency\nDefault unit:  dB \n\n<Carrier>\n float\nPower in the allocated channel (aggregated BW)\nDefault unit:  dBm \n\n<ENDCpos>\n float\nPower in the adjacent channel with higher frequency\nDefault unit:  dB\n\nAvailable Repeated Capabilities:\ninstance: i0, i1, i2, i3, i4, i5, i6, i7, i8, i9, i10, i11, i12, i13, i14, i15, i16, i17, i18, i19, i20, i21, i22, i23, i24, i25, i26, i27, i28, i29, i30, i31, i32\r\n\nRemote-control command(s):\nFETCh:NRSub:MEAS<i>:MEValuation:TRACe:ACLR:ENDC:AVERage?"}, {"Level"=4, "Class Only"=FALSE, "Identifier"="RSCMWXPNRFR1M_ATTR_READ_MULTI_EVAL_MEAS_ACLR_CURRENT_RESULTS", "Descriptive Name"="Read Multi Eval Meas ACLR Current Results", "Data Type"=enum."RawString", "Command"="READ:NRS:MEAS{instance}:MEV:ACLR:CURR?", "Access"=enum."Read Only", "Range Table"="", "Read Callback"="", "Write Callback"="", "Range Callback"="", "Check Callback"="", "Rngtable Callback"="", "Coerce Callback"="", "Supported Models"="", "Instrument Options"="", "Check Status Callback"="", "Flags"=0, "Help"="Returns the relative ACLR values for NR standalone, as displayed in the table below the ACLR diagram. The current values are retrieved.\n\nReturn values:  \n<Reliability>\n decimal\n\n<UTRA2neg>\n float\nACLR for the second UTRA channel with lower frequency\nDefault unit:  dB \n\n<UTRA1neg>\n float\nACLR for the first UTRA channel with lower frequency\nDefault unit:  dB \n\n<NRneg>\n float\nACLR for the first NR channel with lower frequency\nDefault unit:  dB \n\n<Carrier>\n float\nPower in the allocated NR channel\nDefault unit:  dBm \n\n<NRpos>\n float\nACLR for the first NR channel with higher frequency\nDefault unit:  dB \n\n<UTRA1pos>\n float\nACLR for the first UTRA channel with higher frequency\nDefault unit:  dB \n\n<UTRA2pos>\n float\nACLR for the second UTRA channel with higher frequency\nDefault unit:  dB\n\nAvailable Repeated Capabilities:\ninstance: i0, i1, i2, i3, i4, i5, i6, i7, i8, i9, i10, i11, i12, i13, i14, i15, i16, i17, i18, i19, i20, i21, i22, i23, i24, i25, i26, i27, i28, i29, i30, i31, i32\r\n\nRemote-control command(s):\nREAD:NRSub:MEAS<i>:MEValuation:ACLR:CURRent?"}, {"Level"=4, "Class Only"=FALSE, "Identifier"="RSCMWXPNRFR1M_ATTR_READ_MULTI_EVAL_MEAS_ACLR_AVERAGE_RESULTS", "Descriptive Name"="Read Multi Eval Meas ACLR Average Results", "Data Type"=enum."RawString", "Command"="READ:NRS:MEAS{instance}:MEV:ACLR:AVER?", "Access"=enum."Read Only", "Range Table"="", "Read Callback"="", "Write Callback"="", "Range Callback"="", "Check Callback"="", "Rngtable Callback"="", "Coerce Callback"="", "Supported Models"="", "Instrument Options"="", "Check Status Callback"="", "Flags"=0, "Help"="Returns the relative ACLR values for NR standalone, as displayed in the table below the ACLR diagram. The average values are retrieved.\n\nReturn values:  \n<Reliability>\n decimal\n\n<UTRA2neg>\n float\nACLR for the second UTRA channel with lower frequency\nDefault unit:  dB \n\n<UTRA1neg>\n float\nACLR for the first UTRA channel with lower frequency\nDefault unit:  dB \n\n<NRneg>\n float\nACLR for the first NR channel with lower frequency\nDefault unit:  dB \n\n<Carrier>\n float\nPower in the allocated NR channel\nDefault unit:  dBm \n\n<NRpos>\n float\nACLR for the first NR channel with higher frequency\nDefault unit:  dB \n\n<UTRA1pos>\n float\nACLR for the first UTRA channel with higher frequency\nDefault unit:  dB \n\n<UTRA2pos>\n float\nACLR for the second UTRA channel with higher frequency\nDefault unit:  dB\n\nAvailable Repeated Capabilities:\ninstance: i0, i1, i2, i3, i4, i5, i6, i7, i8, i9, i10, i11, i12, i13, i14, i15, i16, i17, i18, i19, i20, i21, i22, i23, i24, i25, i26, i27, i28, i29, i30, i31, i32\r\n\nRemote-control command(s):\nREAD:NRSub:MEAS<i>:MEValuation:ACLR:AVERage?"}, 
